vi "LOOPS.vi"() -> ()   [LabVIEW 2022 SP3]
panel:
  out "Previous Iteration":dbl
  out "Top Iteration":dbl
  out "Numeric":dbl
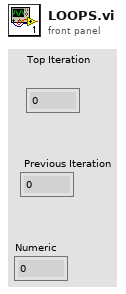
[diagram p1: front panel]
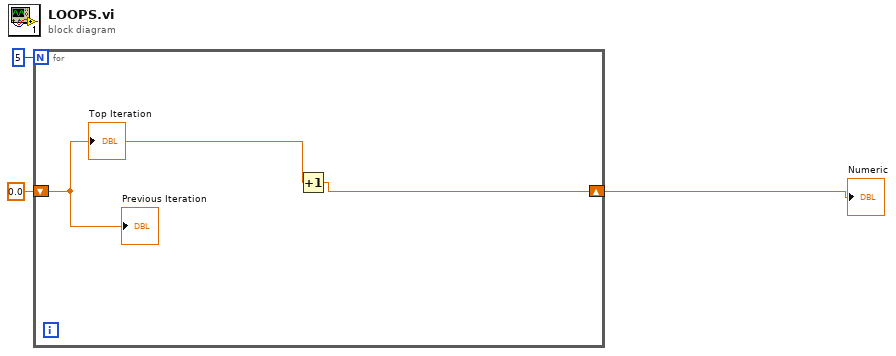
[diagram p0: block diagram]
diagram:
  n1 = for {
    N: 5 -> [_]
    shift-right: [w5] -> w2
    shift-left: 0.0 -> [w4]
    n2 = Increment(x=w4) -> (x+1=w5:dbl)
    "Top Iteration" <- w4
    "Previous Iteration" <- w4
  }
  "Numeric" <- w2
